vi "Set Pump State.vi"(8 "error in (no error)":errorcluster, 10 "Pump State":bool, 11 "Evaporative Cooler in":refnum<class "Evaporative Cooler.lvclass">) -> (0 "error out":errorcluster)   [LabVIEW 2025, in "Evaporative Cooler.lvlib" / "Evaporative Cooler.lvclass"]
doc: "Child classes must override this method to turn the water pump on or off based on the value of the input parameter."
uses:
  Evaporative Cooler.lvclass
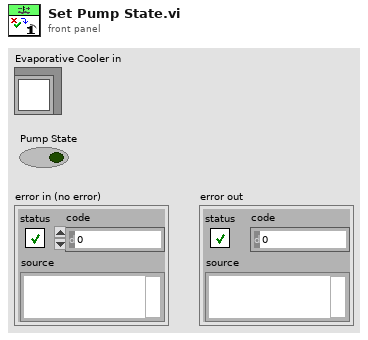
[diagram p1: front panel]
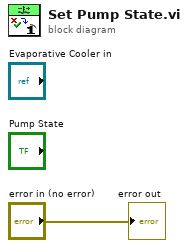
[diagram p0: block diagram]
diagram:
  "error out" <- "error in (no error)"
